vi "IMAQ noise remove.vi"() -> ()   [LabVIEW 2012, in "LightPipes.lvlib"]
uses:
  LightPipes.lvlib
  <vilib>/vision/NI_Vision_Development_Module.lvlib
panel:
  in  "Image Type":T1=7 items=["Grayscale (U8)", "Grayscale (I16)", "Grayscale (SGL)", "Complex (CSG)", "RGB (U32)", "HSL (U32)", "RGB (U64)", "Grayscale (U16)"]
  in  "Noise Value":i32=1
  in  "Stop":bool
  in  "Save":bool
  in  "Noise Remove":bool
  out "Image":T2(plugin-control)
  in  "Input Image Path":path=path "C:/Users/Tri/Documents/Lightpipes/LabView/beam images/OSP Midfield.png"
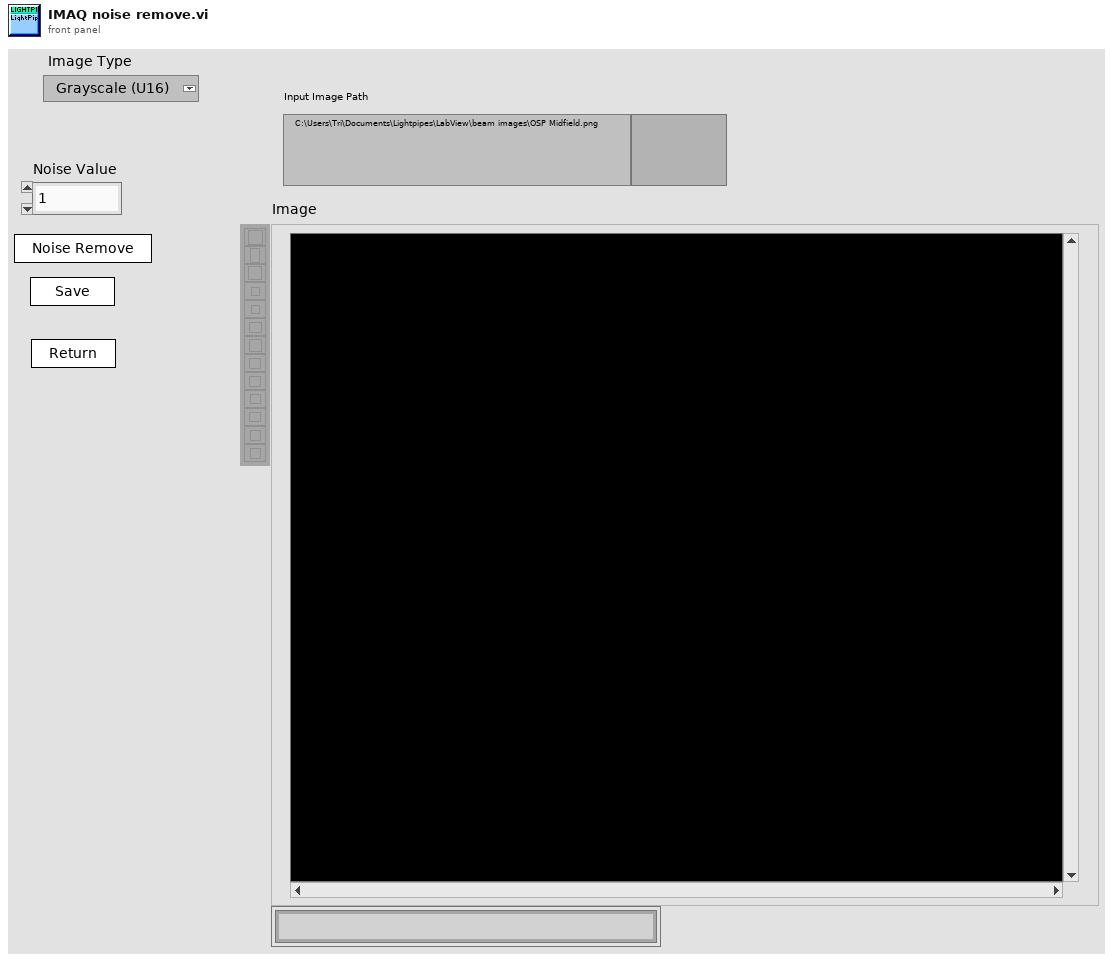
[diagram p1: front panel]
types:
  T1 = typedef "Image Type" = u32
  T2 = typedef "IMAQ Image.ctl" = refnum<image>
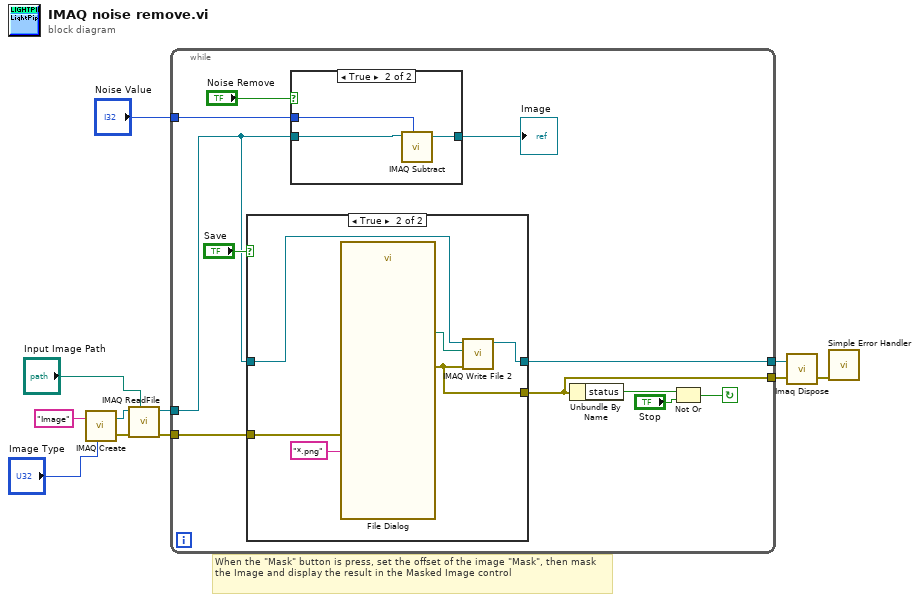
[diagram p0: block diagram]
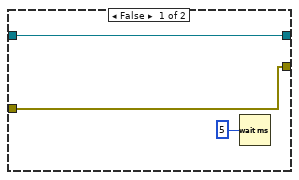
[diagram p3: hidden frame]
diagram:
  # "When the \"Mask\" button is press, set the offset of the image \"Mask\", then mask the Image and display the result in the Masked Image control"
  n1 = call "IMAQ Create"("Image Name"="Image", "Image Type"="Image Type") -> ("New Image"=w7:T2, "error out"=w10:errorcluster)  [unwired: 2 in, 1 out]
  n2 = call "IMAQ ReadFile"("File Path"="Input Image Path", "error in (no error)"=w10, "Image"=w7) -> ("error out"=w9:errorcluster, "Image Out"=w5:T2)  [unwired: 2 in, 5 out]
  n3 = while {
    tunnel: w5 -> [w17]
    tunnel: w9 -> [w14]
    tunnel: [w13] -> w2
    tunnel: [w12] -> w1
    tunnel: "Noise Value" -> [w16]
    stop <- w20 continue-if-true
    n4 = case shown="True" "Save" {
      tunnel: w17 -> [w28 w33]
      tunnel: w14 -> [w27 w32]
      tunnel: [w27 w31] -> w13
      tunnel: [w28 w30] -> w12
      frame False {
        n5 = Wait (ms)(milliseconds to wait=u32 5) -> ()  [unwired: 1 out]
      }
      frame True {
        n6 = call "File Dialog"("error in"=w32, "pattern (all files)"="*.png") -> ("selected path"=w35:path, "error out"=w31:errorcluster)  [unwired: 10 in, 2 out]
        n7 = call-poly "IMAQ Write File 2"("error in (no error)"=w31, "File Path"=w35, "Image"=w33) -> ("Image Out (duplicate)"=w30:T2)  [unwired: 7 in, 1 out]
      }
    }
    n8 = case shown="True" "Noise Remove" {
      tunnel: w17 -> [w23 w26]
      tunnel: w16 -> [_ w25]
      tunnel: [w23 w24] -> w15
      frame False {
      }
      frame True {
        n9 = call "IMAQ Subtract"("Image Src A"=w26, "Constant"=w25) -> ("Image Dst Out"=w24:T2)  [unwired: 5 in, 1 out]
      }
    }
    "Image" <- w15
    n10 = Unbundle By Name(w13) -> ("status"=w22:bool)
    n11 = Not Or(1:"Stop", 2:w22) -> (0:w20:bool)
  }
  n12 = call "Imaq Dispose"("Image"=w1, "error in (no error)"=w2) -> ("error out"=w6:errorcluster)  [unwired: 1 in, 3 out]
  n13 = call <vilib>:"Simple Error Handler.vi"("error in (no error)"=w6) -> ()  [unwired: 1 in, 8 out]
